vi "Check Device Type.vi"(8 "error in (no error)":errorcluster, 9 "Device Type Name":string, 10 "Dual Relay Bricklet in":refnum<class "Dual Relay Bricklet.lvclass">) -> (0 "error out":errorcluster, 1 "correct Device":bool, 2 "Dual Relay Bricklet out":refnum<class "Dual Relay Bricklet.lvclass">)   [LabVIEW 2011, in "Tinkerforge.lvlib" / "Dual Relay Bricklet.lvclass"]
doc: "This VI is the child implementation of \"Check Device Type.vi\" and invokes the device type validation through checking the device name."
uses:
  Dual Relay Bricklet.lvclass
  Device/Device.lvclass
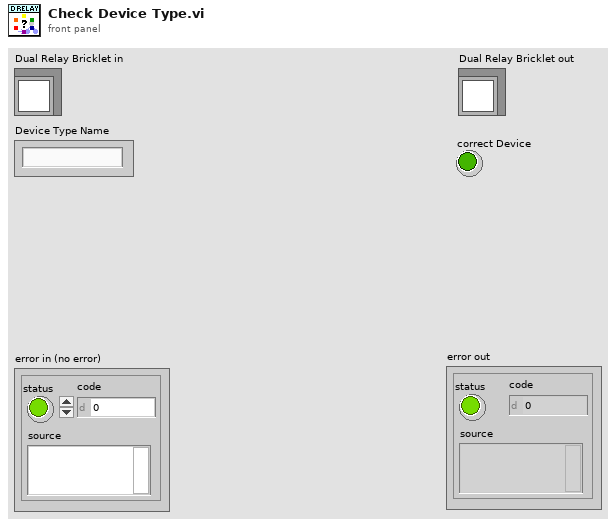
[diagram p1: front panel]
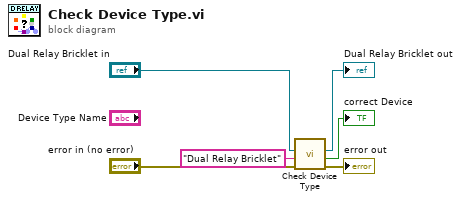
[diagram p0: block diagram]
diagram:
  n1 = call-parent "Check Device Type.vi"("error in (no error)"="error in (no error)", "Device Type Name"="Dual Relay Bricklet", "Device in"="Dual Relay Bricklet in") -> ("error out"=→"error out":errorcluster, "correct Device"=→"correct Device":bool, "Device out"=→"Dual Relay Bricklet out":refnum<class "Dual Relay Bricklet.lvclass">)  [unwired: 6 in]
